vi "WILT Interval Resend.vi"(6 "Send Restart Every? (Sec)":dbl, 9 "Elapsed Time (sec)":dbl, 10 "Station Number in":u32, 11 "Agilent Valve and Switch Locations":T1[](array[typedef])) -> (3 "Sending CMD":bool)   [LabVIEW 2016]
uses:
  Type Definitions/WILT Agilent Channel Definition.ctl
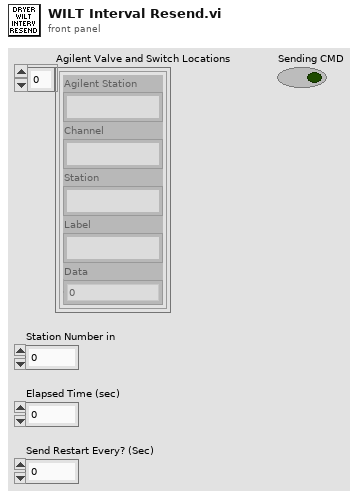
[diagram p1: front panel]
types:
  T1 = typedef "WILT Agilent Channel Definition.ctl" = cluster{"Channel":string, "Station":string, "Label":string, "Agilent Station":string, "Data":dbl}
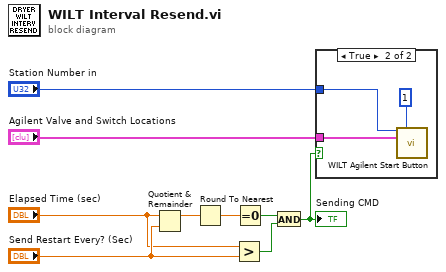
[diagram p0: block diagram]
diagram:
  n1 = Quotient & Remainder(x="Elapsed Time (sec)", y="Send Restart Every? (Sec)") -> (x-y*floor(x/y)=w2:dbl)  [unwired: 1 out]
  n2 = Round To Nearest(number=w2) -> (nearest integer value=w3:dbl)
  n3 = Greater?(x="Elapsed Time (sec)", y="Send Restart Every? (Sec)") -> (0:w1:bool)
  n4 = Equal To 0?(x=w3) -> (x = 0?=w4:bool)
  n5 = And(x=w4, y=w1) -> (x .and. y?=w6:bool)
  "Sending CMD" <- w6
  n6 = case shown="True" w6 {
    tunnel: "Agilent Valve and Switch Locations" -> [_ w11]
    tunnel: "Station Number in" -> [_ w10]
    frame False {
    }
    frame True {
      n7 = call "WILT Agilent Start Button.vi"("Station Number"=w10, "Number Of Cycles"=1, "Agilent Valve and Switch Locations"=w11) -> ()  [unwired: 12 in, 1 out]
    }
  }
